vi "Scan For MFLI.vi"() -> ()   [LabVIEW 2021, in "MFLI Driver.lvclass"]
uses:
  MFLI Driver.lvclass
  <instrlib>/Zurich Instruments LabOne/Public/ziTypeHandle.ctl
  <instrlib>/Zurich Instruments LabOne/Zurich Instruments LabOne.lvlib
panel:
  out "Error Out":errorcluster
  out "Devices":cluster{"Nodes":string, i32}[](array[cluster])
  out "Handle Out":T1 {"Handle" format="0x%08x"; "Conn" format="0x%08x"}
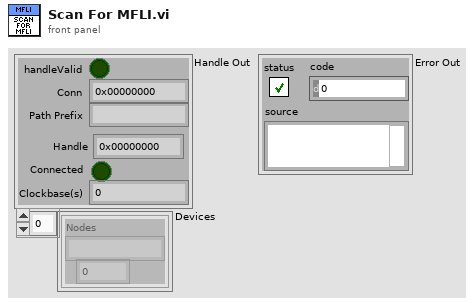
[diagram p1: front panel]
types:
  T1 = typedef "Zurich Instruments LabOne.lvlib/ziTypeHandle.ctl" = cluster{"handleValid":bool, "Conn":u64, "Path Prefix":string, "Handle":u64, "Connected":bool, "Clockbase(s)":dbl}
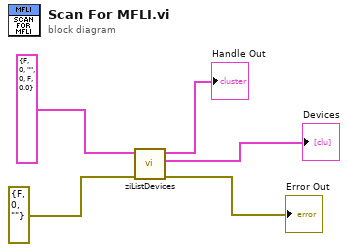
[diagram p0: block diagram]
diagram:
  n1 = call <instrlib>:"ziListDevices.vi"("Error In"=errorcluster {"status"=FALSE, "code"=0, "source"=""}, "Handle In"=T1 {"handleValid"=FALSE, "Conn"=0, "Path Prefix"="", "Handle"=0, "Connected"=FALSE, "Clockbase(s)"=0.0}) -> ("Error Out"=→"Error Out":errorcluster, "Devices"=→"Devices":cluster{"Nodes":string, i32}[], "Handle Out"=→"Handle Out":T1)  [unwired: 3 in]
